vi "InitHardware.vi"(8 "error in (no error)":errorcluster, 11 "ThorLabsCsCamera in":refnum<class "ThorLabsCsCamera.lvclass">) -> (0 "error out":errorcluster, 1 "bit depth":string, 2 "Image Type":T1 items=["Grayscale (U8)", "Grayscale (I16)", "Grayscale (SGL)", "Complex (CSG)", "RGB (U32)", "HSL (U32)", "RGB (U64)", "Grayscale (U16)"], 3 "ThorLabsCsCamera out":refnum<class "ThorLabsCsCamera.lvclass">)   [LabVIEW 2020, in "ThorLabsCsCamera.lvclass"]
uses:
  ThorLabsCsCamera.lvclass
  C:/GEECS/Developers Version/builds/Device builds/ThorlabsCsCamera/Point Grey Camera.lvclass
  Point Grey Camera.lvclass/Point Grey Camera.ctl
  ThorLabsCsCamera.lvclass/ThorLabsCsCamera.ctl
  Read Settings 2.vi
  Write Settings 2.vi
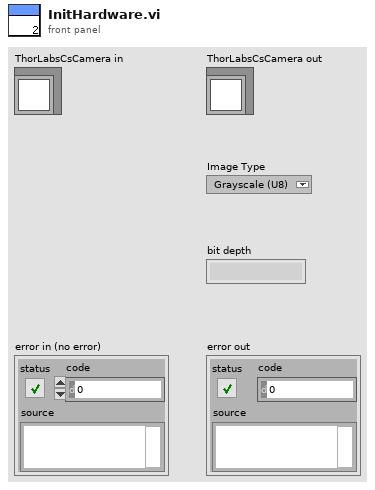
[diagram p1: front panel]
types:
  T1 = typedef "Image Type" = u32
  T2 = typedef "Point Grey Camera.lvclass/SettingsTypdef.ctl" = cluster{"Trigger":T3, "Gain":cluster{"Value":dbl, "Min":dbl, "Max":dbl, "StepSize":dbl, "Tolerance":dbl, "valueactual":dbl}, "Exposure":cluster{"Value":dbl, "Min":dbl, "Max":dbl, "StepSize":dbl, "Tolerance":dbl, "valueactual":dbl}, "Timeout":cluster{"Value":dbl, "Min":dbl, "Max":dbl, "StepSize":dbl, "Tolerance":dbl, "valueactual":dbl}, "LocalSavingPath":path, "Save":T3, "TriggerDelay":cluster{"Value":dbl, "Min":dbl, "Max":dbl, "StepSize":dbl, "Tolerance":dbl, "valueactual":dbl}, "CamSession":string, "ROI":T4, "MaxGUIPixel":cluster{"Value":dbl, "Min":dbl, "Max":dbl, "StepSize":dbl, "Tolerance":dbl, "valueactual":dbl}, "Target":cluster{"X":cluster{"Value":dbl, "Min":dbl, "Max":dbl, "StepSize":dbl, "Tolerance":dbl, "valueactual":dbl}, "Y":cluster{"Value":dbl, "Min":dbl, "Max":dbl, "StepSize":dbl, "Tolerance":dbl, "valueactual":dbl}}, "Analysis":T3, "maxshot#":dbl, "SpatialCalibration":cluster{"Value":dbl, "Min":dbl, "Max":dbl, "StepSize":dbl, "Tolerance":dbl, "valueactual":dbl}, "roistatus":T3, "Lineout":T3, "AnalysisThreshold":cluster{"Value":dbl, "Min":dbl, "Max":dbl, "StepSize":dbl, "Tolerance":dbl, "valueactual":dbl}, "TargetSize":cluster{"X":cluster{"Value":dbl, "Min":dbl, "Max":dbl, "StepSize":dbl, "Tolerance":dbl, "valueactual":dbl}, "Y":cluster{"Value":dbl, "Min":dbl, "Max":dbl, "StepSize":dbl, "Tolerance":dbl, "valueactual":dbl}}, "Simulation":T3, "SpatialCalibrationY":cluster{"Value":dbl, "Min":dbl, "Max":dbl, "StepSize":dbl, "Tolerance":dbl, "valueactual":dbl}, "Target2":cluster{"X":cluster{"Value":dbl, "Min":dbl, "Max":dbl, "StepSize":dbl, "Tolerance":dbl, "valueactual":dbl}, "Y":cluster{"Value":dbl, "Min":dbl, "Max":dbl, "StepSize":dbl, "Tolerance":dbl, "valueactual":dbl}}, "Target2Size":cluster{"X":cluster{"Value":dbl, "Min":dbl, "Max":dbl, "StepSize":dbl, "Tolerance":dbl, "valueactual":dbl}, "Y":cluster{"Value":dbl, "Min":dbl, "Max":dbl, "StepSize":dbl, "Tolerance":dbl, "valueactual":dbl}}, "Crosshair":cluster{"Label1":string, "Label2":string}, "Max2ndMomRadius":cluster{"Value":dbl, "Min":dbl, "Max":dbl, "StepSize":dbl, "Tolerance":dbl, "valueactual":dbl}, "SaveType":T5, "BackgroundPath":path}
  T3 = typedef "OnOffTypeDef.ctl" = enum16{"off", "on"}
  T4 = typedef "ROI_TypDef.ctl" = cluster{"Width":cluster{"Value":dbl, "Min":dbl, "Max":dbl, "StepSize":dbl, "Tolerance":dbl, "valueactual":dbl}, "Height":cluster{"Value":dbl, "Min":dbl, "Max":dbl, "StepSize":dbl, "Tolerance":dbl, "valueactual":dbl}, "OffsetX":cluster{"Value":dbl, "Min":dbl, "Max":dbl, "StepSize":dbl, "Tolerance":dbl, "valueactual":dbl}, "OffsetY":cluster{"Value":dbl, "Min":dbl, "Max":dbl, "StepSize":dbl, "Tolerance":dbl, "valueactual":dbl}}
  T5 = typedef "Image save type.ctl" = enum16{"PNG", "BMP", "JPEG", "TDMS", "hdf5"}
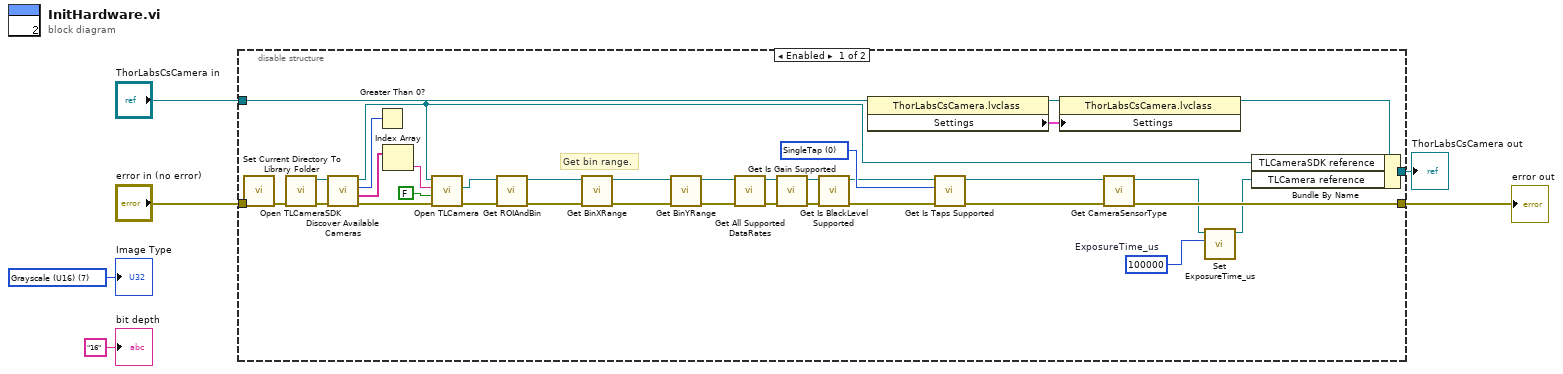
[diagram p0: block diagram]
diagram:
  w1 = T1 7 items=["Grayscale (U8)", "Grayscale (I16)", "Grayscale (SGL)", "Complex (CSG)", "RGB (U32)", "HSL (U32)", "RGB (U64)", "Grayscale (U16)"] ("Image Type")
  n1 = disable-structure shown="Enabled" {
    disable-tunnel: "error in (no error)" -> [w36 w43]
    disable-tunnel: "ThorLabsCsCamera in" -> [w17 w44]
    disable-tunnel: [w11 w44] -> w4
    disable-tunnel: [w10 w43] -> w3
    frame Enabled {
      w7 = u32 100000  # ExposureTime_us
      w28 = 0 items=["SingleTap", "DualTap", "QuadTap"] ("Taps")
      # "Get bin range."
      n2 = call "Set Current Directory To Library Folder.vi"("error in (no error)"=w36) -> ("error out"=w37:errorcluster)  [unwired: 10 in]
      n3 = call "Open TLCameraSDK.vi"("error in (no error)"=w37) -> ("error out"=w39:errorcluster, "TLCameraSDK ref out"=w38:refnum<k24>)  [unwired: 9 in]
      n4 = call "Discover Available Cameras.vi"("error in (no error)"=w39, "TLCameraSDK reference"=w38) -> ("error out"=w14:errorcluster, "Serial Numbers"=w19:string[], "Number of Cameras"=w40:i32, "TLCameraSDK reference out"=w16:refnum<k24>)  [unwired: 6 in]
      n5 = Greater Than 0?(x=w40) -> ()  [unwired: 1 out]
      n6 = Index Array(array=w19) -> (element=w35:string)  [unwired: 1 in]
      n7 = call "Open TLCamera.vi"("error in (no error)"=w14, "isDiagnosticsMessagesEnabled"=FALSE, "Camera serial number"=w35, "TLCameraSDK reference"=w16) -> ("error out"=w33:errorcluster, "TLCamera reference out"=w32:refnum<k24>)  [unwired: 5 in, 1 out]
      n8 = call "Get ROIAndBin.vi"("error in (no error)"=w33, "TLCamera reference in"=w32) -> ("error out"=w31:errorcluster, "TLCamera reference out"=w29:refnum<k24>)  [unwired: 6 in, 2 out]
      n9 = call "Get BinXRange.vi"("error in (no error)"=w31, "TLCamera reference in"=w29) -> ("error out"=w13:errorcluster, "TLCamera reference out"=w30:refnum<k24>)  [unwired: 6 in, 2 out]
      n10 = call "Get BinYRange.vi"("error in (no error)"=w13, "TLCamera reference in"=w30) -> ("error out"=w12:errorcluster, "TLCamera reference out"=w27:refnum<k24>)  [unwired: 6 in, 2 out]
      n11 = call "Get All Supported DataRates.vi"("error in (no error)"=w12, "TLCamera reference"=w27) -> ("error out"=w26:errorcluster, "TLCamera reference out"=w23:refnum<k24>)  [unwired: 7 in, 1 out]
      n12 = call "Get Is Gain Supported.vi"("error in (no error)"=w26, "TLCamera reference in"=w23) -> ("error out"=w22:errorcluster, "TLCamera reference out"=w21:refnum<k24>)  [unwired: 7 in, 1 out]
      n13 = call "Get Is BlackLevel Supported.vi"("error in (no error)"=w22, "TLCamera reference in"=w21) -> ("error out"=w15:errorcluster, "TLCamera reference out"=w20:refnum<k24>)  [unwired: 7 in, 1 out]
      n14 = property class="ThorLabsCsCamera.lvclass"(reference=w17) -> (reference out=w41:refnum<class "ThorLabsCsCamera.lvclass">, "Settings"=w42:T2)  [unwired: 1 in, 1 out]
      n15 = call "Get Is Taps Supported.vi"("error in (no error)"=w15, "Taps"=w28, "TLCamera reference"=w20) -> ("error out"=w25:errorcluster, "TLCamera reference out"=w24:refnum<k24>)  [unwired: 6 in, 1 out]
      n16 = property class="ThorLabsCsCamera.lvclass"(reference=w41, "Settings"=w42) -> (reference out=w18:refnum<class "ThorLabsCsCamera.lvclass">)  [unwired: 1 in, 1 out]
      n17 = call "Get CameraSensorType.vi"("error in (no error)"=w25, "TLCamera reference in"=w24) -> ("error out"=w10:errorcluster, "TLCamera reference out"=w9:refnum<k24>)  [unwired: 7 in, 1 out]
      n18 = call "Set ExposureTime_us.vi"("ExposureTime_us"=w7, "TLCamera reference in"=w9) -> ("TLCamera reference out"=w8:refnum<k24>)  [unwired: 8 in, 1 out]
      n19 = Bundle By Name(cluster=w18, "TLCameraSDK reference"=w16, "TLCamera reference"=w8) -> (w11:refnum<class "ThorLabsCsCamera.lvclass">)
    }
    frame Disabled {
    }
  }
  "ThorLabsCsCamera out" <- w4
  "error out" <- w3
  "Image Type" <- w1
  "bit depth" <- "16" ("bit depth")
